vi "T-Periodic Sawtooth Gate.vi"(4 "Period T":dbl format="%#_4g", 8 "Reversed?":bool, 9 "W":dbl format="%#_4g", 11 "t":dbl format="%#_4g") -> (3 "Sawtooth(t)":dbl format="%#_4g")   [LabVIEW 2021, in "Math.lvlib"]
uses:
  Math.lvlib
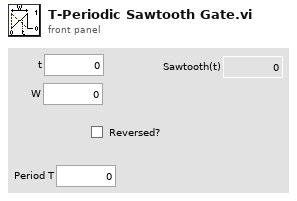
[diagram p1: front panel]
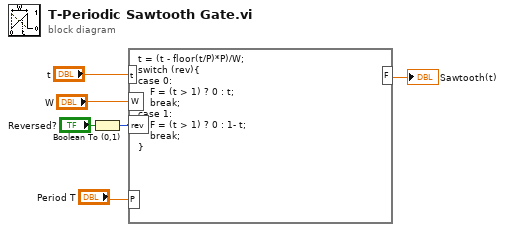
[diagram p0: block diagram]
diagram:
  n1 = Boolean To (0,1)(Boolean="Reversed?") -> (0, 1=w2:i16)
  n2 = formula code="t = (t - floor(t/P)*P)/W;\nswitch (rev){\ncase 0:\n    F = (t > 1) ? 0 : t;\n    break;\ncase 1:\n    F = (t > 1) ? 0 : 1- t;\n    break;\n}"("t"="t", "W"="W", "P"="Period T", "rev"=w2) -> ("F"=→"Sawtooth(t)":dbl)
